vi "Search for Project Files.vi"(0 "Search Directory":path, 5 "Recursive Search? (F)":bool, 11 "error in (no error)":errorcluster) -> (4 "Project Files":T1, 15 "error out":errorcluster)   [LabVIEW 2016, in "Digital.lvlib"]
uses:
  Digital.lvlib
  <vilib>/ErrorRing/Error Ring.xnode
  Type Definitions/Project Files.ctl
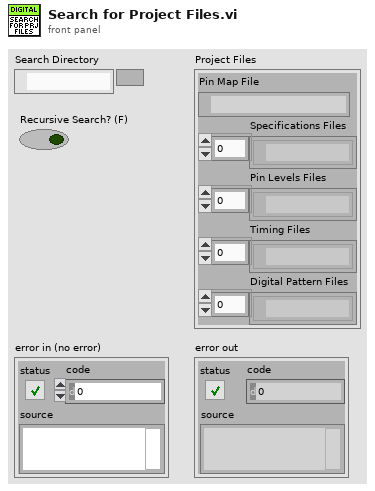
[diagram p1: front panel]
types:
  T1 = typedef "Digital.lvlib/Project Files.ctl" = cluster{"Pin Map File":path, "Specifications Files":path[], "Pin Levels Files":path[], "Timing Files":path[], "Digital Pattern Files":path[]}
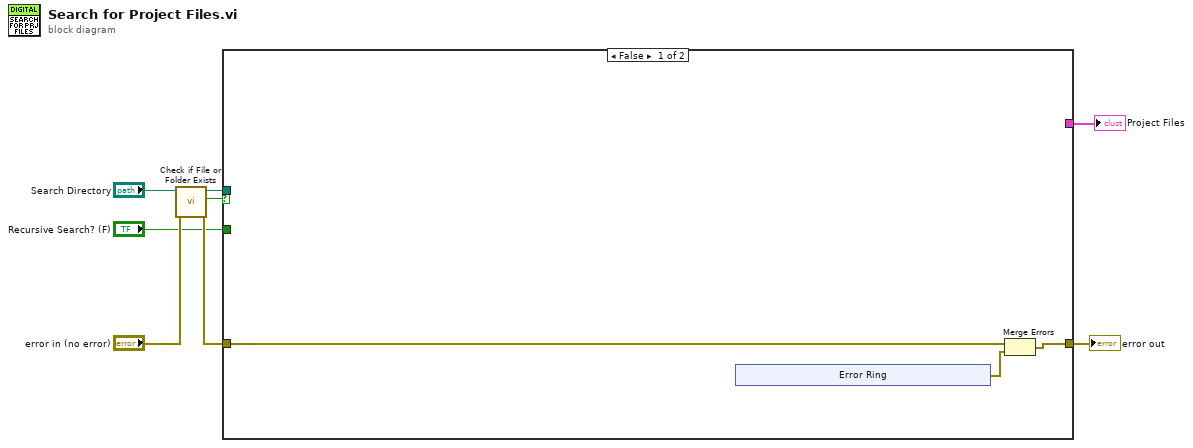
[diagram p0: block diagram]
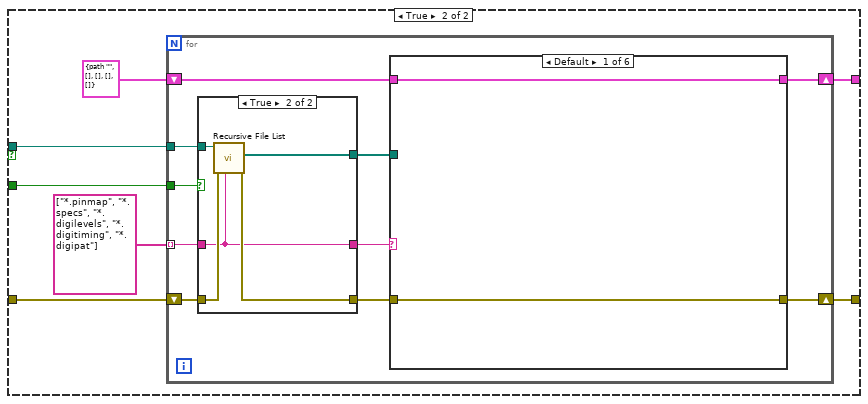
[diagram p2: hidden frame]
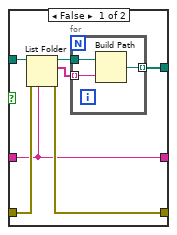
[diagram p3: hidden frame]
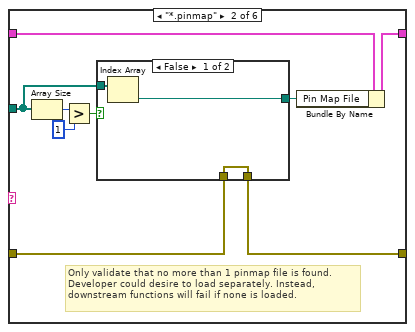
[diagram p4: hidden frame]
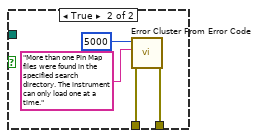
[diagram p5: hidden frame]
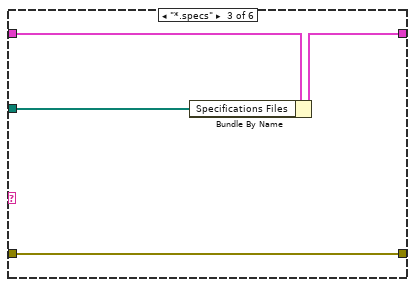
[diagram p6: hidden frame]
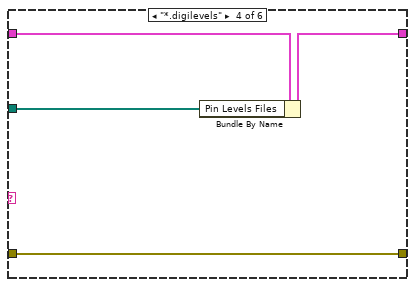
[diagram p7: hidden frame]
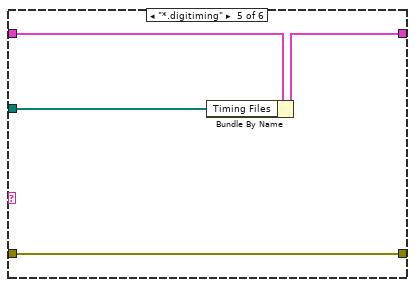
[diagram p8: hidden frame]
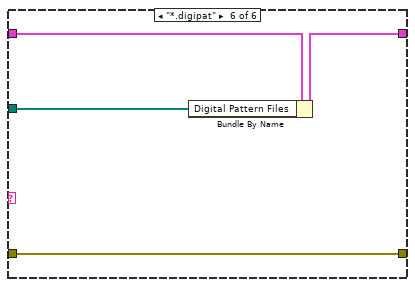
[diagram p9: hidden frame]
diagram:
  n1 = call <vilib>:"Check if File or Folder Exists.vi"("error in (no error)"="error in (no error)", "path"="Search Directory") -> ("error out"=w7:errorcluster, "file or folder exists?"=w4:bool, "dup path"=w3:path)  [unwired: 7 in]
  n2 = case shown="False" w4 {
    tunnel: w7 -> [w11 w22]
    tunnel: [w10 w17] -> w6
    tunnel: w3 -> [_ w21]
    tunnel: "Recursive Search? (F)" -> [_ w20]
    tunnel: [_ w16] -> w1
    frame False {
      n3 = xnode "Error Ring"() -> ("error out"=w9:errorcluster)
      n4 = Merge Errors(w11, w9) -> (w10:errorcluster)
    }
    frame True {
      n5 = for {
        tunnel: w21 -> [w31]
        tunnel: w20 -> [w30]
        tunnel: string[] ["*.pinmap", "*.specs", "*.digilevels", "*.digitiming", "*.digipat"] -> [w29] mode=indexing
        shift-right: [w26] -> w17
        shift-left: w22 -> [w32]
        shift-right: [w24] -> w16
        shift-left: T1 {"Pin Map File"=path "", "Specifications Files"=[], "Pin Levels Files"=[], "Timing Files"=[], "Digital Pattern Files"=[]} ("Project Files") -> [w25]
        n6 = case shown="True" w30 {
          tunnel: w31 -> [w37 w45]
          tunnel: w32 -> [w39 w47]
          tunnel: [w38 w46] -> w27
          tunnel: w29 -> [w33 w43]
          tunnel: [w34 w44] -> w23
          tunnel: [w33 w43] -> w28
          frame False {
            n7 = List Folder(path=w37, pattern=w33, error in=w39) -> (path out=w36:path, filenames=w35:string[], error out=w38:errorcluster)  [unwired: 2 out]
            n8 = for {
              tunnel: w36 -> [w42]
              tunnel: w35 -> [w41] mode=indexing
              tunnel: [w40] -> w34 mode=indexing
              n9 = Build Path(base path=w42, name or relative path=w41) -> (appended path=w40:path)
            }
          }
          frame True {
            n10 = call <vilib>:"Recursive File List.vi"("pattern"=w43, "error in (no error)"=w47, "Folder Path"=w45) -> ("error out"=w46:errorcluster, "All Files in Dir"=w44:path[])  [unwired: 4 in, 3 out]
          }
        }
        n11 = case shown="Default" w28 {
          tunnel: w27 -> [w48 w51 w68 w72 w76 w80]
          tunnel: [w48 w52 w68 w72 w76 w80] -> w26
          tunnel: w25 -> [w49 w58 w69 w73 w77 w81]
          tunnel: [w49 w57 w67 w71 w75 w79] -> w24
          tunnel: w23 -> [_ w53 w66 w70 w74 w78]
          frame Default {
          }
          frame "*.pinmap" {
            # "Only validate that no more than 1 pinmap file is found. Developer could desire to load separately. Instead, downstream functions will fail if none is loaded."
            n12 = Array Size(array=w53) -> (size(s)=w55:i32)
            n13 = Greater?(x=w55, y=1) -> (0:w56:bool)
            n14 = case shown="False" w56 {
              tunnel: [w61 _] -> w50
              tunnel: w53 -> [w60 _]
              tunnel: w51 -> [w59 w63]
              tunnel: [w59 w62] -> w52
              frame False {
                n15 = Index Array(array=w60) -> (element=w61:path)  [unwired: 1 in]
              }
              frame True {
                n16 = call <vilib>:"Error Cluster From Error Code.vi"("error in (no error)"=w63, "error message (\"\")"="More than one Pin Map files were found in the specified search directory. The instrument can only load one at a time.", "error code (0)"=5000) -> ("error out"=w62:errorcluster)  [unwired: 6 in]
              }
            }
            n17 = Bundle By Name(cluster=w58, "Pin Map File"=w50) -> (w57:T1)
          }
          frame "*.specs" {
            n18 = Bundle By Name(cluster=w69, "Specifications Files"=w66) -> (w67:T1)
          }
          frame "*.digilevels" {
            n19 = Bundle By Name(cluster=w73, "Pin Levels Files"=w70) -> (w71:T1)
          }
          frame "*.digitiming" {
            n20 = Bundle By Name(cluster=w77, "Timing Files"=w74) -> (w75:T1)
          }
          frame "*.digipat" {
            n21 = Bundle By Name(cluster=w81, "Digital Pattern Files"=w78) -> (w79:T1)
          }
        }
      }
    }
  }
  "error out" <- w6
  "Project Files" <- w1
